vi "HW_Stream_raw_data_enq.vi"(8 "error in":errorcluster, 9 "Queue in":refnum<queue>, 10 "Data flow controls":T2, 11 "VISA resource name in":refnum<visa-resource-name>) -> (0 "error out":errorcluster, 1 "Data frame":T1, 2 "Data flow controls out":T2, 3 "VISA resource name out":refnum<visa-resource-name>, 4 "Queue out":refnum<queue>)   [LabVIEW 2016]
uses:
  <vilib>/Instr/_visa.llb/VISA Flush IO Buffer Mask.ctl
panel:
  out "Timestamp":timestamp
  out "Read buffer":string
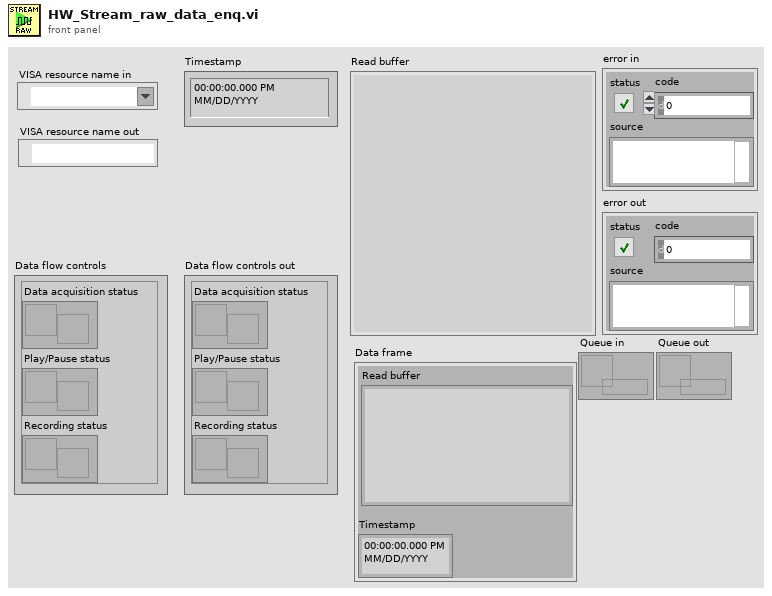
[diagram p1: front panel]
types:
  T1 = cluster{"Read buffer":string, "Timestamp":timestamp}
  T2 = cluster{"Data acquisition status":refnum<notifier>, "Play/Pause status":refnum<notifier>, "Recording status":refnum<notifier>}
  T3 = typedef "VISA Flush IO Buffer Mask.ctl" = u16
  T4 = cluster{"result string":string, "seconds since 1Jan1904":timestamp}
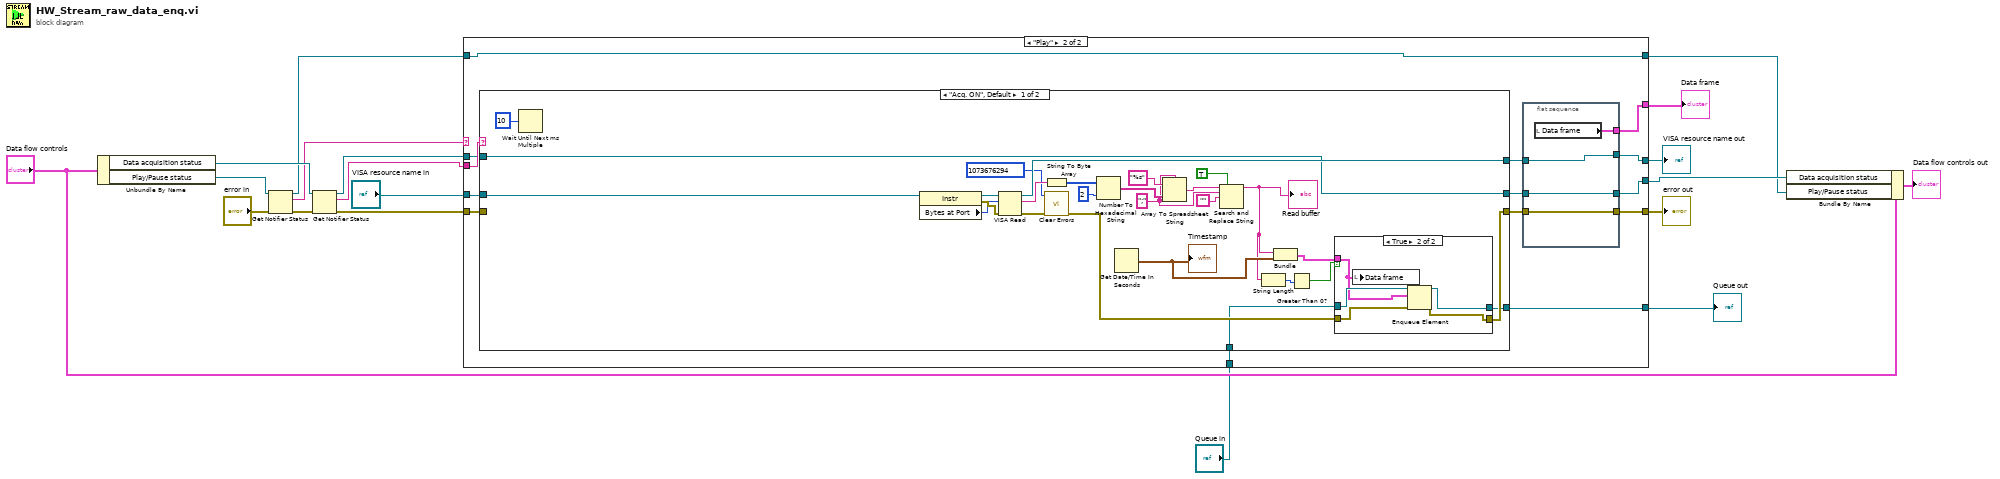
[diagram p0: block diagram]
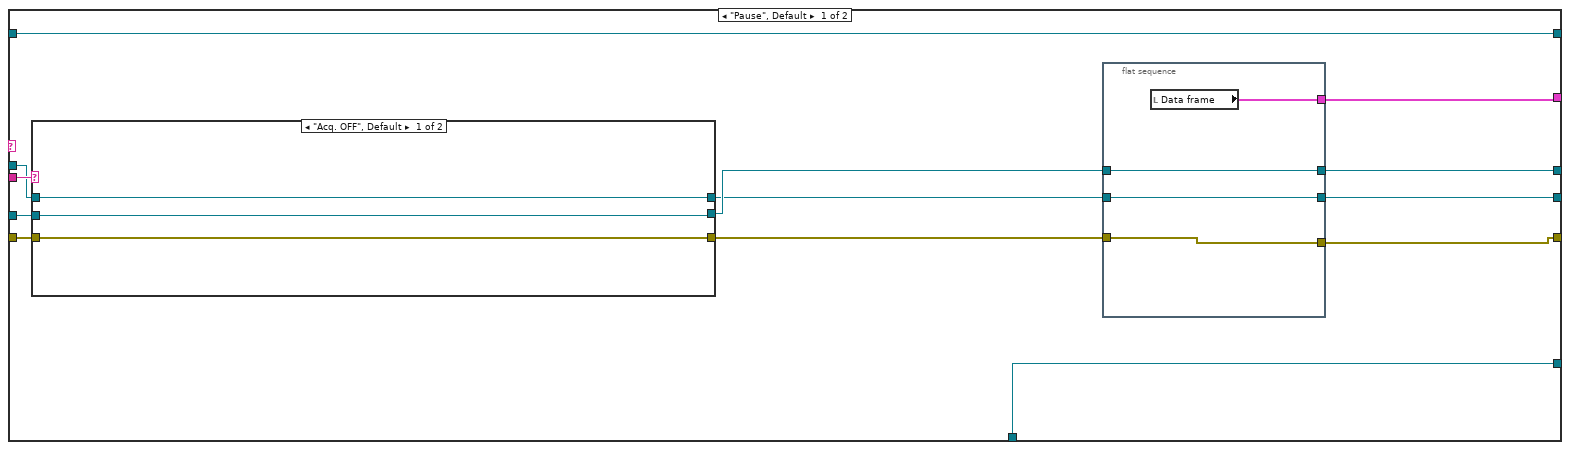
[diagram p2: hidden frame]
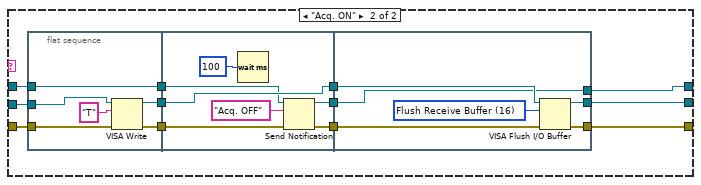
[diagram p3: hidden frame]
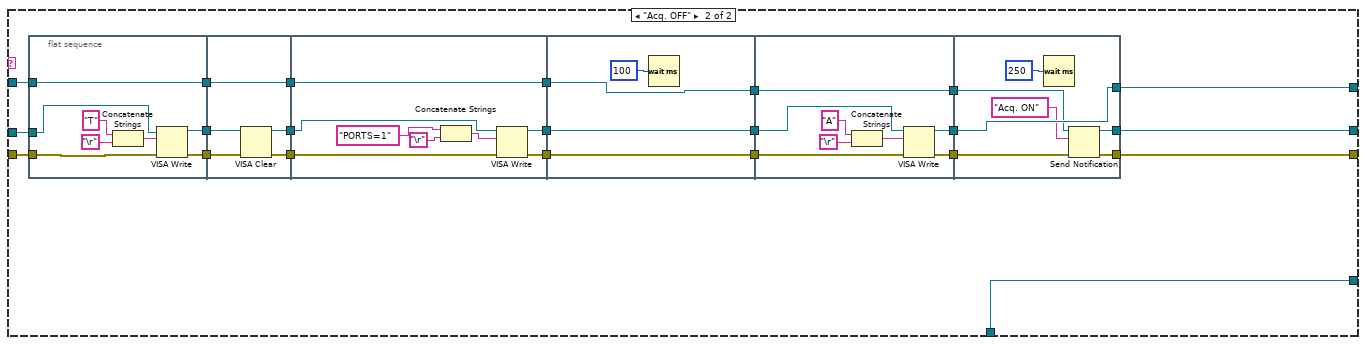
[diagram p5: hidden frame]
diagram:
  n1 = Unbundle By Name("Data flow controls") -> ("Data acquisition status"=w17:refnum<notifier>, "Play/Pause status"=w16:refnum<notifier>)
  n2 = Get Notifier Status(notifier=w16, error in (no error)="error in") -> (notifier out=w11:refnum<notifier>, current notification=w15:string, error out=w12:errorcluster)  [unwired: 2 out]
  n3 = Get Notifier Status(notifier=w17, error in (no error)=w12) -> (notifier out=w10:refnum<notifier>, current notification=w14:string, error out=w5:errorcluster)  [unwired: 2 out]
  n4 = case shown="\"Play\"" w15 {
    tunnel: [w26 w78] -> w18
    tunnel: "VISA resource name in" -> [w32 w84]
    tunnel: w14 -> [w31 w82]
    tunnel: w11 -> [w29 w80]
    tunnel: w10 -> [w30 w81]
    tunnel: [w24 w76] -> w8
    tunnel: [w29 w80] -> w7
    tunnel: w5 -> [w28 w83]
    tunnel: [w22 w74] -> w4
    tunnel: [w27 w79] -> w3
    tunnel: "Queue in" -> [w20 w72]
    tunnel: [w20 w71] -> w1
    frame "Pause", Default {
      n5 = case shown="\"Acq. OFF\", Default" w31 {
        tunnel: w32 -> [w39 w49]
        tunnel: [w39 w48] -> w25
        tunnel: w30 -> [w38 w42]
        tunnel: [w38 w41] -> w23
        tunnel: w28 -> [w37 w45]
        tunnel: [w37 w44] -> w21
        frame "Acq. OFF", Default {
        }
        frame "Acq. ON" {
          n6 = flat-sequence {
            tunnel: w49 -> [w57]
            tunnel: [w56] -> w51
            tunnel: [w55] -> w50
            tunnel: w45 -> [w53]
            tunnel: [w52] -> w43
            tunnel: w42 -> [w52]
            tunnel: w51 -> [w63]
            tunnel: w50 -> [w62]
            tunnel: [w63] -> w47
            tunnel: [w61] -> w46
            tunnel: w43 -> [w59]
            tunnel: [w58] -> w40
            tunnel: [w68] -> w48
            tunnel: w47 -> [w69]
            tunnel: w46 -> [w70]
            tunnel: [w66] -> w44
            tunnel: [w65] -> w41
            tunnel: w40 -> [w65]
            frame #0 {
              n7 = VISA Write(VISA resource name=w57, write buffer="T", error in (no error)=w53) -> (VISA resource name out=w56:refnum<visa-resource-name>, error out=w55:errorcluster)  [unwired: 1 out]
            }
            frame #1 {
              n8 = Wait (ms)(milliseconds to wait=u32 100) -> ()  [unwired: 1 out]
              n9 = Send Notification(notification="Acq. OFF", notifier=w59, error in (no error)=w62) -> (notifier out=w58:refnum<notifier>, error out=w61:errorcluster)
            }
            frame #2 {
              w67 = T3 16 items=["Flush Receive Buffer"=16, "Write Transmit Buffer to Device"=32, "Flush Receive Buffer (No I/O)"=64, "Flush Transmit Buffer"=128] ("Mask")
              n10 = VISA Flush I/O Buffer(VISA resource name=w69, mask (16)=w67, error in (no error)=w70) -> (VISA resource name out=w68:refnum<visa-resource-name>, error out=w66:errorcluster)
            }
          }
        }
      }
      n11 = flat-sequence {
        tunnel: [w36] -> w27
        tunnel: [w35] -> w26
        tunnel: w25 -> [w35]
        tunnel: [w34] -> w24
        tunnel: w23 -> [w34]
        tunnel: [w33] -> w22
        tunnel: w21 -> [w33]
        frame #0 {
          n12 = local read "Data frame"() -> (w36:T1)
        }
      }
    }
    frame "Play" {
      n13 = case shown="\"Acq. ON\", Default" w82 {
        tunnel: w84 -> [w115 w142]
        tunnel: [w111 w141] -> w77
        tunnel: [w91 w140] -> w73
        tunnel: w83 -> [_ w131]
        tunnel: w81 -> [w98 w125]
        tunnel: [w98 w124] -> w75
        tunnel: w72 -> [w90 w123]
        tunnel: [w89 w123] -> w71
        frame "Acq. ON", Default {
          w105 = ";" ("delimiter (Tab)")
          n14 = Wait Until Next ms Multiple(millisecond multiple=u32 10) -> ()  [unwired: 1 out]
          n15 = property class="Instr"(reference=w115) -> (reference out=w114:refnum<visa-resource-name>, error out=w113:errorcluster, "Bytes at Port"=w112:u32)  [unwired: 1 in]
          n16 = VISA Read(VISA resource name=w114, byte count=w112, error in (no error)=w113) -> (VISA resource name out=w111:refnum<visa-resource-name>, read buffer=w103:string, error out=w100:errorcluster)  [unwired: 1 out]
          n17 = String To Byte Array(string=w103) -> (unsigned byte array=w110:u8[])
          n18 = call <vilib>:"Clear Errors.vi"("error in (no error)"=w100, "specific error code to clear (0: all)"=1073676294) -> ("error out"=w92:errorcluster)  [unwired: 4 in, 1 out]
          n19 = Number To Hexadecimal String(1:i16 2 ("width (-)"), 2:w110) -> (0:w108:string[])
          n20 = Get Date/Time In Seconds ("Current time")() -> (seconds since 1Jan1904=w97:timestamp)
          "Timestamp" <- w97
          n21 = Array To Spreadsheet String(delimiter (Tab)=w105, array=w108, 3:"%s" ("format string")) -> (spreadsheet string=w106:string)
          n22 = Search and Replace String(replace all?=TRUE ("replace all? (F)"), input string=w106, search string=w105, replace string="") -> (result string=w95:string)  [unwired: 4 in, 3 out]
          "Read buffer" <- w95
          n23 = String Length(string=w95) -> (length=w94:i32)
          n24 = Bundle("result string"=w95, "seconds since 1Jan1904"=w97) -> (w96:T4)  [unwired: 1 in]
          n25 = Greater Than 0?(x=w94) -> (x > 0?=w93:bool)
          n26 = case shown="True" w93 {
            tunnel: w96 -> [_ w121]
            tunnel: w92 -> [w117 w119]
            tunnel: [w117 w118] -> w91
            tunnel: w90 -> [w116 w122]
            tunnel: [w116 w120] -> w89
            frame False {
            }
            frame True {
              n27 = local write "Data frame"(w121) -> ()
              n28 = Enqueue Element(queue=w122, element=w121, error in (no error)=w119) -> (queue out=w120:refnum<queue>, error out=w118:errorcluster)  [unwired: 1 in, 1 out]
            }
          }
        }
        frame "Acq. OFF" {
          n29 = flat-sequence {
            tunnel: w142 -> [w151]
            tunnel: [w152] -> w139
            tunnel: [w150] -> w138
            tunnel: w131 -> [w146]
            tunnel: [w145] -> w126
            tunnel: w125 -> [w145]
            tunnel: [w157] -> w133
            tunnel: [w156] -> w132
            tunnel: w138 -> [w155]
            tunnel: w139 -> [w154]
            tunnel: [w153] -> w127
            tunnel: w126 -> [w153]
            tunnel: w133 -> [w163]
            tunnel: [w162] -> w137
            tunnel: w132 -> [w161]
            tunnel: [w160] -> w136
            tunnel: [w158] -> w128
            tunnel: w127 -> [w158]
            tunnel: [w169] -> w135
            tunnel: [w168] -> w134
            tunnel: w136 -> [w168]
            tunnel: w137 -> [w169]
            tunnel: [w166] -> w129
            tunnel: w128 -> [w166]
            tunnel: [w172] -> w144
            tunnel: [w171] -> w143
            tunnel: w135 -> [w174]
            tunnel: w134 -> [w173]
            tunnel: [w170] -> w130
            tunnel: w129 -> [w170]
            tunnel: [w181] -> w140
            tunnel: w144 -> [w182]
            tunnel: w143 -> [w183]
            tunnel: [w183] -> w141
            tunnel: w130 -> [w180]
            tunnel: [w179] -> w124
            frame #0 {
              n30 = Concatenate Strings("T" ("write buffer"), "\r") -> (w147:string)
              n31 = VISA Write(VISA resource name=w151, write buffer=w147, error in (no error)=w146) -> (VISA resource name out=w152:refnum<visa-resource-name>, error out=w150:errorcluster)  [unwired: 1 out]
            }
            frame #1 {
              n32 = VISA Clear(VISA resource name=w154, error in (no error)=w155) -> (VISA resource name out=w157:refnum<visa-resource-name>, error out=w156:errorcluster)
            }
            frame #2 {
              n33 = Concatenate Strings("PORTS=1" ("write buffer"), "\r") -> (w164:string)
              n34 = VISA Write(VISA resource name=w163, write buffer=w164, error in (no error)=w161) -> (VISA resource name out=w162:refnum<visa-resource-name>, error out=w160:errorcluster)  [unwired: 1 out]
            }
            frame #3 {
              n35 = Wait (ms)(milliseconds to wait=u32 100) -> ()  [unwired: 1 out]
            }
            frame #4 {
              n36 = Concatenate Strings("A" ("write buffer"), "\r") -> (w175:string)
              n37 = VISA Write(VISA resource name=w174, write buffer=w175, error in (no error)=w173) -> (VISA resource name out=w171:refnum<visa-resource-name>, error out=w172:errorcluster)  [unwired: 1 out]
            }
            frame #5 {
              n38 = Wait (ms)(milliseconds to wait=u32 250) -> ()  [unwired: 1 out]
              n39 = Send Notification(notification="Acq. ON", notifier=w180, error in (no error)=w182) -> (notifier out=w179:refnum<notifier>, error out=w181:errorcluster)
            }
          }
        }
      }
      n40 = flat-sequence {
        tunnel: [w88] -> w79
        tunnel: [w87] -> w78
        tunnel: w77 -> [w87]
        tunnel: [w86] -> w76
        tunnel: w75 -> [w86]
        tunnel: [w85] -> w74
        tunnel: w73 -> [w85]
        frame #0 {
          n41 = local read "Data frame"() -> (w88:T1)
        }
      }
    }
  }
  "VISA resource name out" <- w18
  "error out" <- w4
  "Data frame" <- w3
  "Queue out" <- w1
  n42 = Bundle By Name(cluster="Data flow controls", "Data acquisition status"=w8, "Play/Pause status"=w7) -> (→"Data flow controls out":T2)
